vi "combinations.vi"(11 "nr of resistors":i32) -> (3 "2D boolean table":bool[][](array[boolean]))   [LabVIEW 2017]
panel:
  out "possibilities":i32
  out "all combinations":string[](array[string])
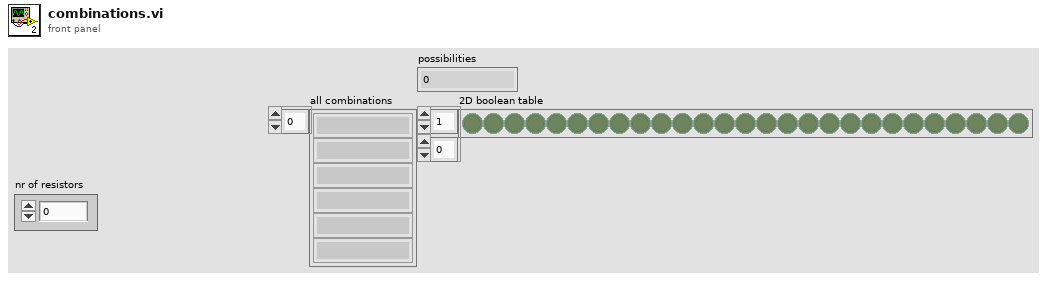
[diagram p1: front panel]
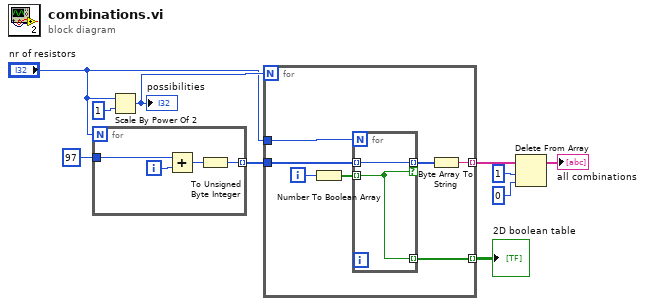
[diagram p0: block diagram]
diagram:
  n1 = for {
    N: "nr of resistors" -> [_]
    tunnel: 97 ("nr of resistors") -> [w14]
    tunnel: [w11] -> w8 mode=indexing
    i -> [w13]
    n2 = Add(x=w14, y=w13) -> (x+y=w12:i32)
    n3 = To Unsigned Byte Integer(number=w12) -> (unsigned 8bit integer=w11:u8)
  }
  n4 = Scale By Power Of 2(n="nr of resistors", x=1 ("nr of resistors")) -> (x*2^n=w7:i32)
  "possibilities" <- w7
  n5 = for {
    N: w7 -> [_]
    tunnel: "nr of resistors" -> [w18]
    tunnel: w8 -> [w21]
    tunnel: [w17] -> w6 mode=indexing
    tunnel: [w15] -> w2 mode=indexing
    i -> [w20]
    n6 = Number To Boolean Array(number=w20) -> (Boolean array=w19:bool[])
    n7 = for {
      N: w18 -> [_]
      tunnel: w21 -> [w23] mode=indexing
      tunnel: w19 -> [w22] mode=indexing
      tunnel: [w23] -> w16 mode=indexing if=w22
      tunnel: [w22] -> w15 mode=indexing
    }
    n8 = Byte Array To String(unsigned byte array=w16) -> (string=w17:string)
  }
  "2D boolean table" <- w2
  n9 = Delete From Array(array=w6, length=1 ("longueur"), index=0 ("indice")) -> (array with subset deleted=→"all combinations":string[])  [unwired: 1 out]
